vi "DemodSubCar_14443A.vi"(8 "error in (no error)":errorcluster, 11 "output array":u8[](array[numeric])) -> (0 "error out":errorcluster, 3 "Array":u8[](array[numeric]))   [LabVIEW 2019]
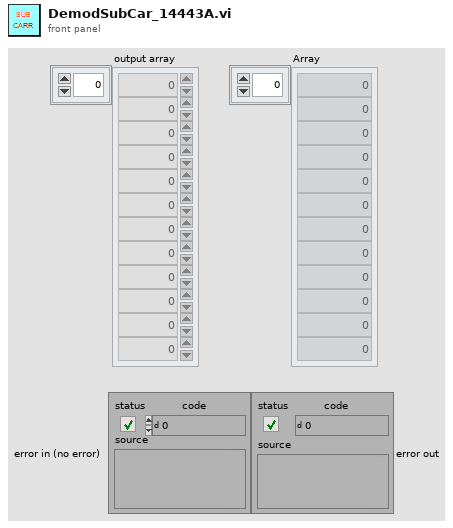
[diagram p1: front panel]
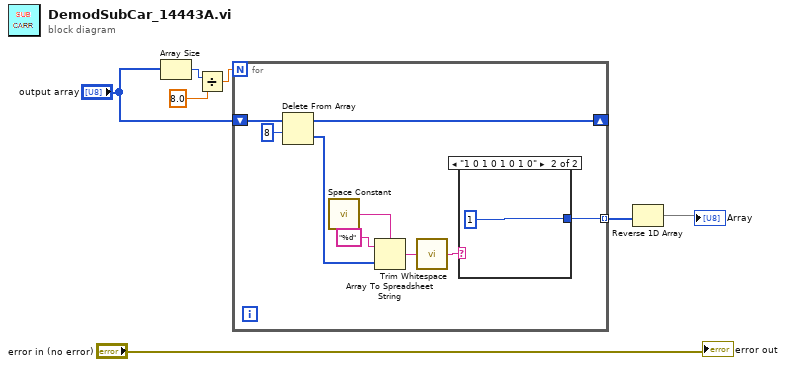
[diagram p0: block diagram]
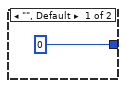
[diagram p2: hidden frame]
diagram:
  n1 = Array Size(array="output array") -> (size(s)=w7:i32)
  n2 = Divide(x=w7, y=8.0) -> (x/y=w6:dbl)
  n3 = for {
    N: w6 -> [_]
    shift-right: [w15] -> _
    shift-left: "output array" -> [w16]
    tunnel: [w9] -> w3 mode=indexing
    n4 = Delete From Array(array=w16, length=8) -> (deleted portion=w8:u8[], array with subset deleted=w15:u8[])  [unwired: 1 in]
    n5 = call <vilib>:"Space Constant.vi"() -> ("String"=w10:string)
    n6 = Array To Spreadsheet String(delimiter (Tab)=w10, array=w8, 3:"%d" ("format string")) -> (spreadsheet string=w12:string)
    n7 = call <vilib>:"Trim Whitespace.vi"("string"=w12) -> ("trimmed string"=w11:string)  [unwired: 1 in]
    n8 = case shown="\"1 0 1 0 1 0 1 0\"" w11 {
      tunnel: [u8 0 u8 1] -> w9
      frame "", Default {
      }
      frame "1 0 1 0 1 0 1 0" {
      }
    }
  }
  n9 = Reverse 1D Array(array=w3) -> (reversed array=→"Array":u8[])
  "error out" <- "error in (no error)"
